vi "LPD_String to Enum.vi"(0 "Variant (Enum)":variant, 5 "Lookup String (for error reporting)":string, 7 "Enum Value String":string, 11 "error in (no error)":errorcluster) -> (4 "Value (typecast back to enum)":u16, 15 "error out":errorcluster)   [LabVIEW 2009]
doc: "Searches for Enum Value String in the enum that is input as a Variant and returns the Value as a U16.\n\n<B>Typecast the Value output</B> back to the same enum as was input at Variant outside of this VI.\n\n\nAuthor: Mike Schultz\n\n\nLogicPD, Inc\nwww.logicpd.com"
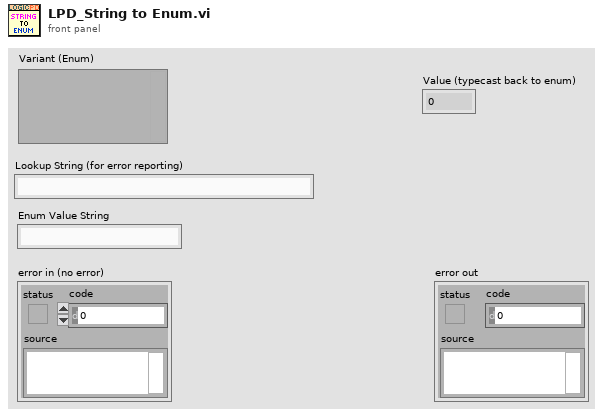
[diagram p1: front panel]
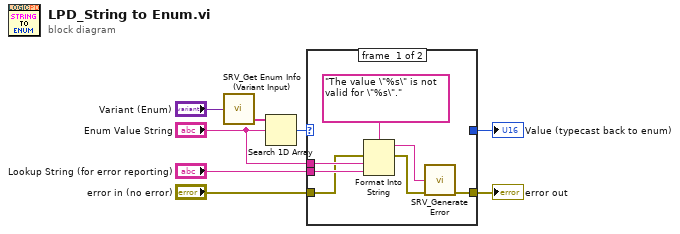
[diagram p0: block diagram]
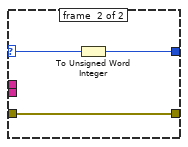
[diagram p2: hidden frame]
diagram:
  n1 = call "SRV_Get Enum Info (Variant Input).vi"("Variant (Enum)"="Variant (Enum)") -> ("Enum Strings"=w2:string[])  [unwired: 4 in, 2 out]
  n2 = Search 1D Array(1D array=w2, element="Enum Value String") -> (index of element=w3:i32)  [unwired: 1 in]
  n3 = case shown="-1" w3 {
    selector: w3 -> [_ w18]
    tunnel: "error in (no error)" -> [w10 w17]
    tunnel: "Enum Value String" -> [w14 _]
    tunnel: [w12 w17] -> w6
    tunnel: "Lookup String (for error reporting)" -> [w13 _]
    tunnel: [_ w16] -> w8
    frame #0 {
      n4 = Format Into String(format string="The value \"%s\" is not valid for \"%s\".", error in=w10, w14, w13) -> (resulting string=w9:string, error out=w11:errorcluster)  [unwired: 1 in]
      n5 = call "SRV_Generate Error.vi"("Message"=w9, "error in (no error)"=w11) -> ("error out"=w12:errorcluster)  [unwired: 13 in]
    }
    frame #1 {
      n6 = To Unsigned Word Integer(number=w18) -> (unsigned 16bit integer=w16:u16)
    }
  }
  "Value (typecast back to enum)" <- w8
  "error out" <- w6
